vi "T_step_initial_Kelvinox.vi"(3 "Current T Setpoint (K)":dbl) -> ()   [LabVIEW 2019]
uses:
  Monitors/Utility/Monitor Communication/Kelvinox/Kelvinox_Control.ctl
  Global/Global Variables/global.vi
  Instrument_Setup.vi
  Global/Global Variables/Data_Display_global.vi
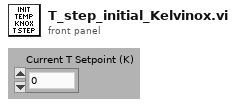
[diagram p1: front panel]
types:
  T1 = typedef "Kelvinox_Status.ctl" = cluster{"V1":bool, "V2":bool, "Dump":u16, "V4":bool, "V5":bool, "V9":bool, "P1":dbl, "P2":dbl, "P3":dbl, "P4":dbl, "P5":dbl, "Turbo":bool, "Forepump":bool, "speed":dbl, "Sorb":dbl, "1K Pot":dbl, "Still":dbl, "Cold\nPlate":dbl, "MC":dbl, "4K":dbl, "Sample":dbl, "T-Setpoint":dbl, "MC Heater":dbl, "Still Heater":dbl, "Sorb Heater":dbl, "T Control active":bool, "Sorb Res":dbl, "1K Pot Res":dbl, "Still Res":dbl, "Cold Plate Res":dbl, "MC Res":dbl, "4K Res":dbl, "Sample Res":dbl, "Ramping":bool, "Sample Res 2":dbl, "Sample 2":dbl}
  T2 = typedef "Kelvinox_Control.ctl" = cluster{"T-Setpoint-Manual":dbl, "Rate (K/min)":dbl, "Change T Control Status":bool, "Emergency Stop":bool, "Set Setpoint":bool}
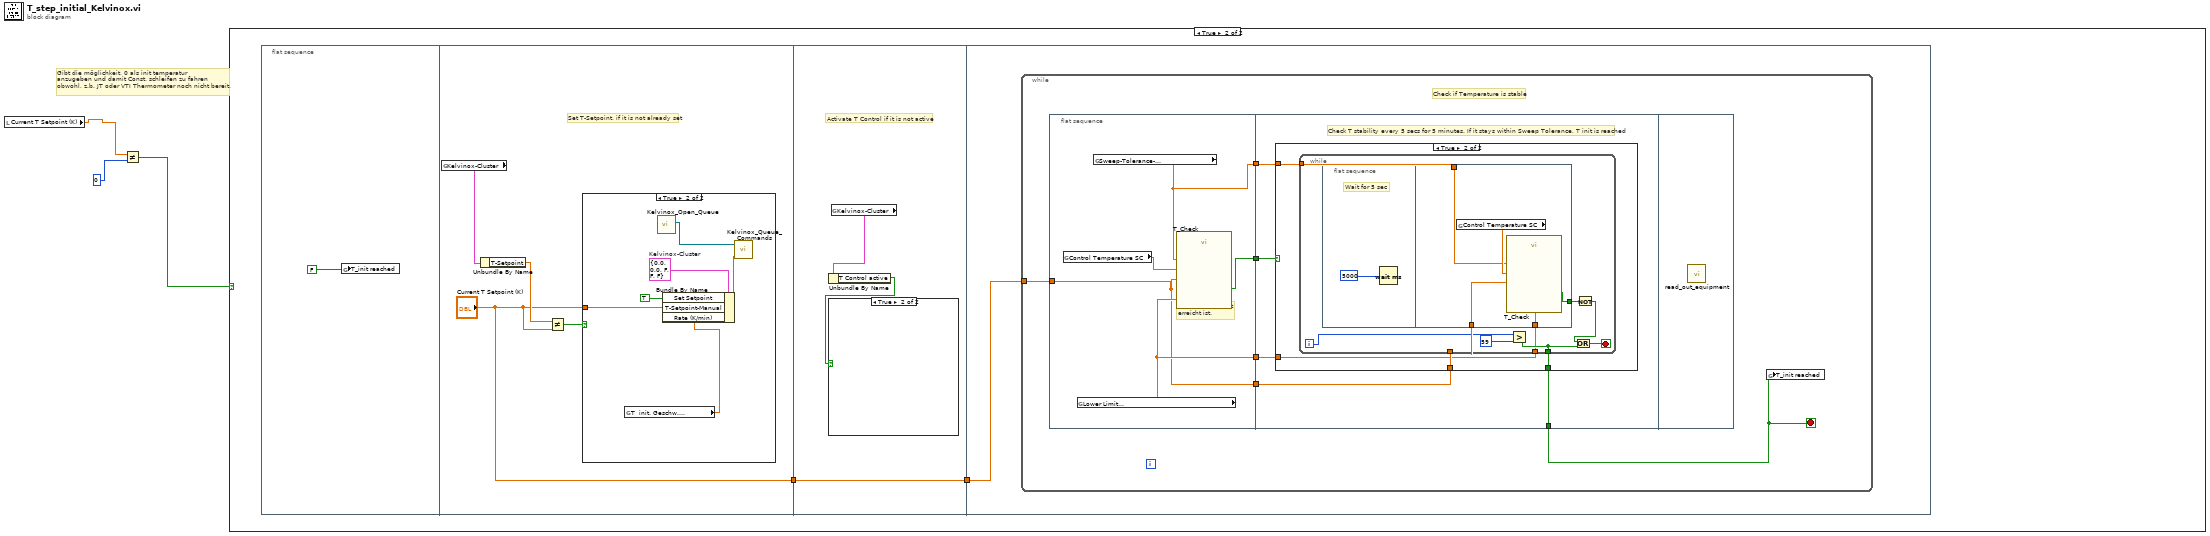
[diagram p0: block diagram]
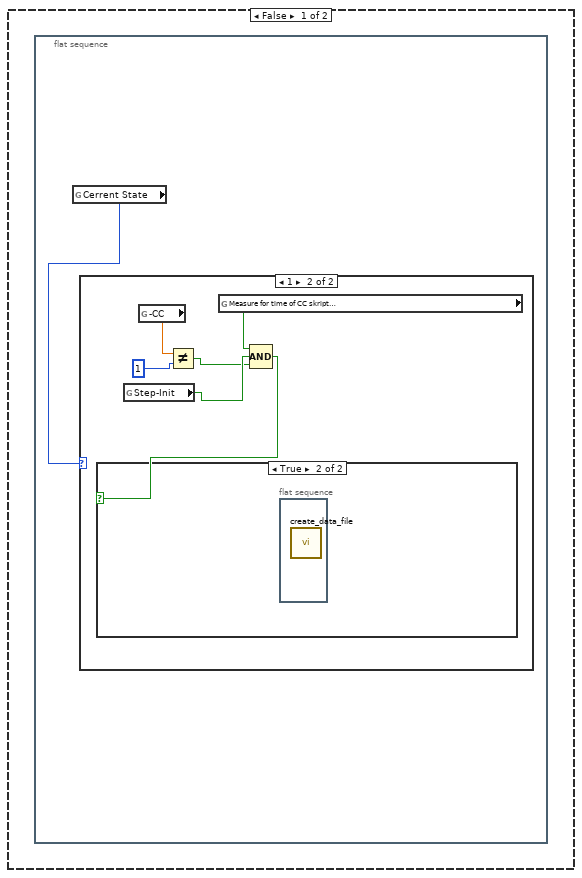
[diagram p2: hidden frame]
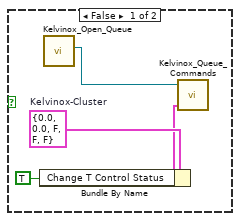
[diagram p6: hidden frame]
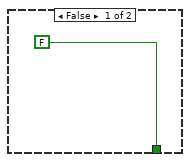
[diagram p7: hidden frame]
diagram:
  # "Gibt die möglichkeit, 0 als init temperatur \nanzugeben und damit Const. schleifen zu fahren\nobwohl, z.b. JT oder VTI Thermometer noch nicht bereit."
  n1 = local read "Current T Setpoint (K)"() -> (w1:dbl)
  n2 = Not Equal?(x=w1, y=0) -> (x != y?=w2:bool)
  n3 = case shown="True" w2 {
    frame False {
      n4 = flat-sequence {
        frame #0 {
          n5 = global read "global.vi" "Cerrent State"() -> (w4:i32)
          n6 = case shown="1" w4 {
            frame 0, Default {
            }
            frame 1 {
              n7 = global read "global.vi" "Step-Init"() -> (w8:bool)
              n8 = global read "global.vi" "-CC"() -> (w7:dbl)
              n9 = Not Equal?(x=w7, y=1) -> (x != y?=w5:bool)
              n10 = global read "Instrument_Setup.vi" "Measure for time of CC skript\nat each field step point"() -> (w10:bool)
              n11 = Compound Arithmetic op=AND(w10, w8, w5) -> (w9:bool)
              n12 = case shown="True" w9 {
                frame False {
                }
                frame True {
                  n13 = flat-sequence {
                    frame #0 {
                      n14 = call "create_data_file.vi"() -> ()  [unwired: 3 in]
                    }
                  }
                }
              }
            }
          }
        }
      }
    }
    frame True {
      n15 = flat-sequence {
        tunnel: ["Current T Setpoint (K)"] -> w11
        tunnel: [w24] -> w12
        tunnel: w11 -> [w24]
        tunnel: w12 -> [w31]
        frame #0 {
          n16 = global write "Data_Display_global.vi" "T_init reached"(FALSE) -> ()
        }
        frame #1 {
          # "Set T-Setpoint, if it is not already set"
          n17 = global read "Data_Display_global.vi" "Kelvinox-Cluster"() -> (w17:T1)
          n18 = Unbundle By Name(w17) -> ("T-Setpoint"=w15:dbl)
          n19 = Not Equal?(x=w15, y="Current T Setpoint (K)") -> (x != y?=w16:bool)
          n20 = case shown="True" w16 {
            tunnel: "Current T Setpoint (K)" -> [_ w19]
            frame False {
            }
            frame True {
              w22 = T2 {"T-Setpoint-Manual"=0.0, "Rate (K/min)"=0.0, "Change T Control Status"=FALSE, "Emergency Stop"=FALSE, "Set Setpoint"=FALSE}  # Kelvinox-Cluster
              n21 = global read "global.vi" "T  init. Geschw. \n(K/min)"() -> (w18:dbl)
              n22 = call "Kelvinox_Open_Queue.vi"() -> ("queue out"=w23:refnum<queue>)  [unwired: 10 in, 1 out]
              n23 = Bundle By Name(cluster=w22, "Set Setpoint"=TRUE, "T-Setpoint-Manual"=w19, "Rate (K/min)"=w18) -> (w21:T2)
              n24 = call "Kelvinox_Queue_Commands.vi"("Control"=w21, "Queue"=w23) -> ()  [unwired: 1 in, 1 out]
            }
          }
        }
        frame #2 {
          # "Activate T Control if it is not active"
          n25 = global read "Data_Display_global.vi" "Kelvinox-Cluster"() -> (w26:T1)
          n26 = Unbundle By Name(w26) -> ("T Control active"=w25:bool)
          n27 = case shown="True" w25 {
            frame False {
              w29 = T2 {"T-Setpoint-Manual"=0.0, "Rate (K/min)"=0.0, "Change T Control Status"=FALSE, "Emergency Stop"=FALSE, "Set Setpoint"=FALSE}  # Kelvinox-Cluster
              n28 = Bundle By Name(cluster=w29, "Change T Control Status"=TRUE) -> (w28:T2)
              n29 = call "Kelvinox_Open_Queue.vi"() -> ("queue out"=w30:refnum<queue>)  [unwired: 10 in, 1 out]
              n30 = call "Kelvinox_Queue_Commands.vi"("Control"=w28, "Queue"=w30) -> ()  [unwired: 1 in, 1 out]
            }
            frame True {
            }
          }
        }
        frame #3 {
          n31 = while {
            tunnel: w31 -> [w32]
            stop <- w37 stop-if-true
            # "Check if Temperature is stable"
            n32 = flat-sequence {
              tunnel: [w41] -> w36
              tunnel: [w38] -> w35
              tunnel: [w40] -> w34
              tunnel: [w39] -> w33
              tunnel: w32 -> [w38]
              tunnel: [w44] -> w37
              tunnel: w36 -> [w47]
              tunnel: w35 -> [w46]
              tunnel: w34 -> [w45]
              tunnel: w33 -> [w43]
              frame #0 {
                # "Check ob T_target\nerreicht ist."
                n33 = global read "Data_Display_global.vi" "Control Temperature SC"() -> (w42:dbl)
                n34 = global read "Instrument_Setup.vi" "Lower Limit\nSweep-Tolerance-\nTemperature (K)"() -> (w39:dbl)
                n35 = global read "Instrument_Setup.vi" "Sweep-Tolerance-\nTemperature (%)"() -> (w40:dbl)
                n36 = call "T_Check.vi"("Lower Limit Sweep\nTolerance (K)"=w39, "T_target (K)"=w38, "Sweep\nTolerance %"=w40, "T_in"=w42) -> ("= T target"=w41:bool)
              }
              frame #1 {
                # "Check T stability every 5 secs for 5 minutes. If it stays within Sweep Tolerance, T init is reached"
                n37 = case shown="True" w47 {
                  tunnel: w46 -> [_ w52]
                  tunnel: w45 -> [_ w51]
                  tunnel: [FALSE w50] -> w44
                  tunnel: w43 -> [_ w49]
                  frame False {
                  }
                  frame True {
                    n38 = while {
                      tunnel: w52 -> [w61]
                      tunnel: w51 -> [w60]
                      tunnel: [w54] -> w50
                      tunnel: w49 -> [w53]
                      i -> [w57]
                      stop <- w58 stop-if-true
                      n39 = flat-sequence {
                        tunnel: [w66] -> w59
                        tunnel: w61 -> [w65]
                        tunnel: w60 -> [w64]
                        tunnel: w53 -> [w63]
                        frame #0 {
                          # "Wait for 5 sec"
                          n40 = Wait (ms)(milliseconds to wait=5000) -> ()  [unwired: 1 out]
                        }
                        frame #1 {
                          n41 = global read "Data_Display_global.vi" "Control Temperature SC"() -> (w67:dbl)
                          n42 = call "T_Check.vi"("Lower Limit Sweep\nTolerance (K)"=w63, "T_target (K)"=w65, "Sweep\nTolerance %"=w64, "T_in"=w67) -> ("= T target"=w66:bool)
                        }
                      }
                      n43 = Greater?(x=w57, y=59) -> (0:w54:bool)
                      n44 = Not(x=w59) -> (.not. x?=w55:bool)
                      n45 = Or(x=w55, y=w54) -> (x .or. y?=w58:bool)
                    }
                  }
                }
              }
              frame #2 {
                n46 = call "read_out_equipment.vi"() -> ()  [unwired: 1 in]
              }
            }
            n47 = global write "Data_Display_global.vi" "T_init reached"(w37) -> ()
          }
        }
      }
    }
  }
